vi "Test Pass if Unexpected Element Not in Map.vi"(8 "error in (no error)":errorcluster, 11 "LUnit Test Case V2 Test Double In":refnum<class "Test Case Test Double.lvclass">) -> (0 "error out":errorcluster, 3 "LUnit Test Case V2 Test Double Out":refnum<class "Test Case Test Double.lvclass">)   [LabVIEW 2020, in "Test Case Test Double.lvclass"]
uses:
  Test Case Test Double.lvclass
  C:/git/astemes-lunit/source/LUnit Test Case.lvclass
  source/Core/LUnit Test Case/LUnit Test Case.lvclass/LUnit Test Case.ctl
  4916146d-4c63-44d0-ad26-501d88454236.vi
  source/Core/LUnit Test Case/Assertions/Fail If.vi
  source/Core/LUnit Test Case/Private/Append Pass Result.vi
  source/Core/LUnit Test Case/Private/Append Fail Result.vi
  source/Core/LUnit Test Case/Private/Run In UI.vi
  <vilib>/Utility/error.llb/Clear Errors.vi
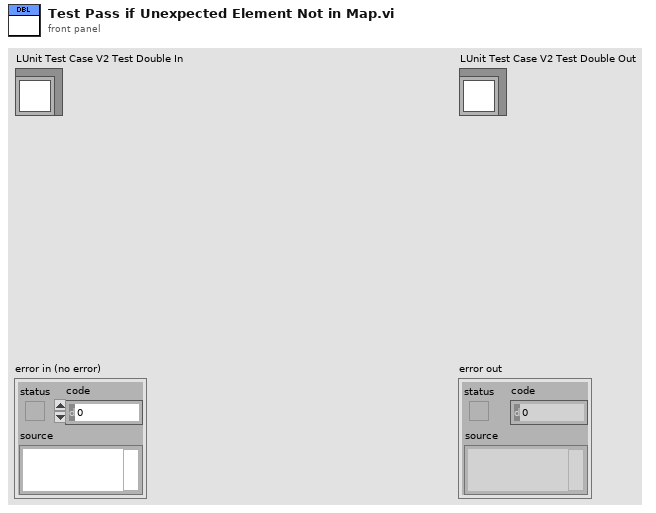
[diagram p1: front panel]
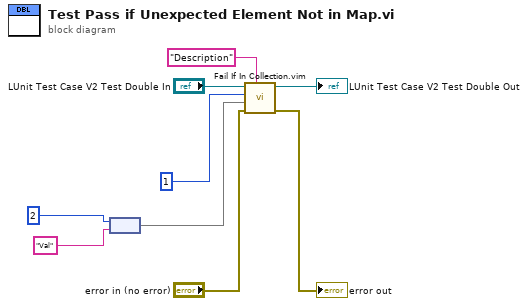
[diagram p0: block diagram]
diagram:
  n1 = node(2, "Val") -> (w1:map{i32, string})
  n2 = call "Fail If In Collection.vim"("Description"="Description", "error in (no error)"="error in (no error)", "Collection"=w1, "Element"=1, "LUnit Test Case In"="LUnit Test Case V2 Test Double In") -> ("error out"=→"error out":errorcluster, "LUnit Test Case Out"=→"LUnit Test Case V2 Test Double Out":refnum<class "Test Case Test Double.lvclass">)  [unwired: 5 in]
